vi "run.add_video.vi"(8 "error in":errorcluster, 11 "Client in":refnum<class "Client.lvclass">) -> (0 "error out":errorcluster, 3 "Client out":refnum<class "Client.lvclass">)   [LabVIEW 2020, in "Client.lvclass"]
doc: "Associates a video with the run under a named reference and returns a handle to the updated run."
uses:
  Client.lvclass
  Client.lvclass/Client.ctl
  client.lvlib
panel:
  out "out_run out":i32
  in  "rid":string
  in  "ref_name":string
  in  "video_rid":string
  in  "out_run":i32
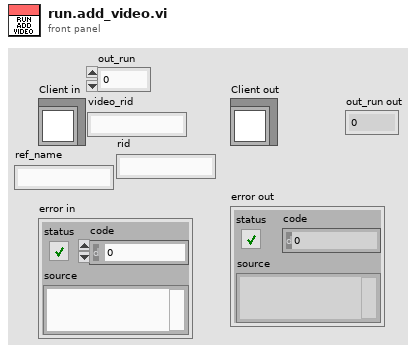
[diagram p1: front panel]
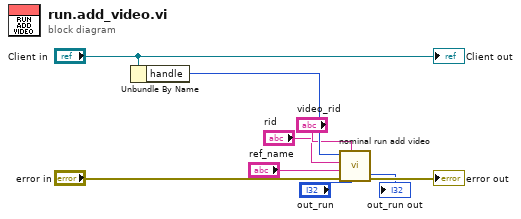
[diagram p0: block diagram]
diagram:
  n1 = Unbundle By Name("Client in") -> ("handle"=w7:i32)
  n2 = call "nominal run add video.vi"("out_run"="out_run", "video_rid"="video_rid", "error in (no error)"="error in", "ref_name"="ref_name", "rid"="rid", "client"=w7) -> ("error out"=→"error out":errorcluster, "out_run out"=→"out_run out":i32)  [unwired: 3 in, 1 out]
  "Client out" <- "Client in"
